vi "Power Output Find Pad Values.vi"(11 "Test Parameters":T1={"Stimulus"={"Frequency Type"=enum."Band Edges", "Frequency Ranges"=[], "TX 1 Frequency (MHz)"={"Min"=0.0, "Max"=0.0}, "TX 2 Frequency (MHz)"={"Min"=0.0, "Max"=0.0}, "RX Frequency (MHz)"={"Min"=0.0, "Max"=0.0}, "Pad Model Number"="", "Pad Serial Number"="", "Pad Values"=[]}, "Measurement"={"DUT Port"=enum."Port 1", "Direction"=0, "Frequency Step Size"=0}, "Display"={"Frequency"={"Min"=-1.0, "Max"=-1.0}, "Power"={"Min"=-1, "Max"=-1}}, "Limit"={"Min Power (dBm)"=44.0}, "Calibration"={"Calibrated?"=FALSE}} {"Measurement"."Frequency Step Size" items=["0.2", "0.4", "1.0", "2.0", "4.0"]; "Measurement"."Direction" items=["Reverse", "Forward", "Auxiliary"]}) -> (2 "Values Present?":bool, 3 "Pad Values Out":dbl[][](array[numeric]))   [LabVIEW 2011]
uses:
  TypeDefs/Power Output Test Parameters.ctl
  TypeDefs/Power Output Stimulus Parameters.ctl
  TypeDefs/Power Output Measurement Parameters.ctl
  BPIMCore EXT/HW IO/DUTport.ctl
  BPIMCore EXT/HW IO/MeasMode.ctl
  BPIMCore EXT/HW IO/PIM Sweep Step Size.ctl
  TypeDefs/Power Output Display Parameters.ctl
  TypeDefs/Power Output Limit Parameters.ctl
  TypeDefs/Power Output Calibration State.ctl
  Summitek EXT/OpenG EXT/array/array.llb/Filter 1D Array with Scalar (DBL)__ogtk.vi
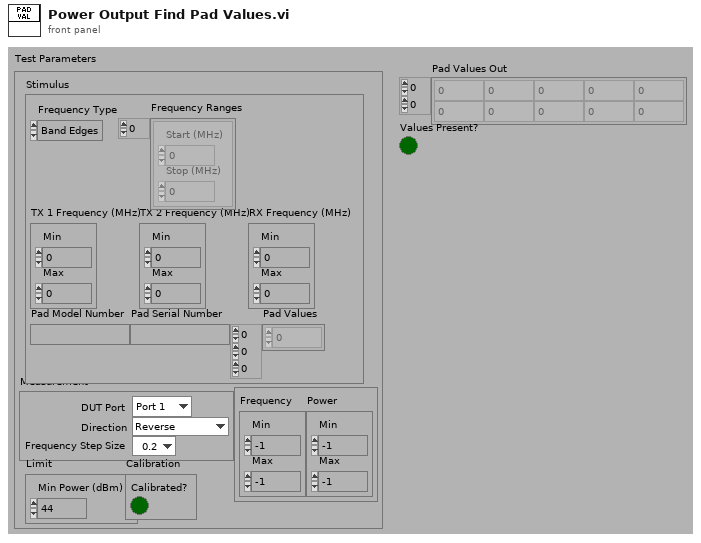
[diagram p1: front panel]
types:
  T1 = typedef "Power Output Test Parameters.ctl" = cluster{"Stimulus":T2, "Measurement":T3, "Display":T7, "Limit":T8, "Calibration":T9}
  T2 = typedef "Power Output Stimulus Parameters.ctl" = cluster{"Frequency Type":enum16{"Band Edges", "Custom"}, "Frequency Ranges":cluster{"Start (MHz)":dbl, "Stop (MHz)":dbl}[], "TX 1 Frequency (MHz)":cluster{"Min":dbl, "Max":dbl}, "TX 2 Frequency (MHz)":cluster{"Min":dbl, "Max":dbl}, "RX Frequency (MHz)":cluster{"Min":dbl, "Max":dbl}, "Pad Model Number":string, "Pad Serial Number":string, "Pad Values":dbl[][][]}
  T3 = typedef "Power Output Measurement Parameters.ctl" = cluster{"DUT Port":T4, "Direction":T5, "Frequency Step Size":T6}
  T4 = typedef "DUTport.ctl" = enum16{"Port 1", "Port 2"}
  T5 = typedef "MeasMode.ctl" = u16
  T6 = typedef "PIM Sweep Step Size.ctl" = u16
  T7 = typedef "Power Output Display Parameters.ctl" = cluster{"Frequency":cluster{"Min":dbl, "Max":dbl}, "Power":cluster{"Min":i32, "Max":i32}}
  T8 = typedef "Power Output Limit Parameters.ctl" = cluster{"Min Power (dBm)":dbl}
  T9 = typedef "Power Output Calibration State.ctl" = cluster{"Calibrated?":bool}
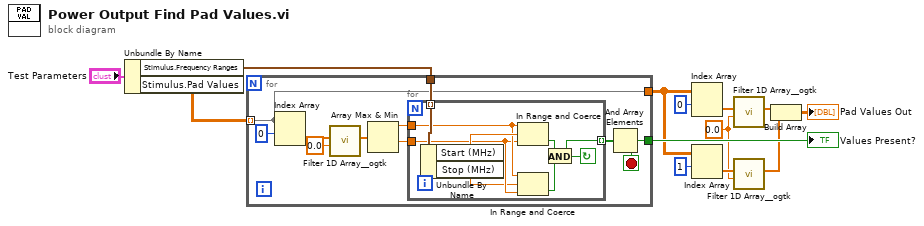
[diagram p0: block diagram]
diagram:
  w3 = 0.0
  n1 = Unbundle By Name("Test Parameters") -> ("Stimulus.Frequency Ranges"=w11:cluster{"Start (MHz)":dbl, "Stop (MHz)":dbl}[], "Stimulus.Pad Values"=w10:dbl[][][])
  n2 = for {
    tunnel: w10 -> [w14] mode=indexing
    tunnel: w11 -> [w22]
    tunnel: [w20] -> w13
    tunnel: [w14] -> w1
    stop <- w20 stop-if-true
    n3 = Index Array(array=w14, index (row)=0 ("disabled index (col)")) -> (element=w15:dbl[])  [unwired: 1 in]
    n4 = call-poly "Filter 1D Array__ogtk.vi"("items to filter"=0.0, "array"=w15) -> ("filtered array"=w16:dbl[])  [unwired: 4 in, 1 out]
    n5 = Array Max & Min(array=w16) -> (max value=w19:dbl, min value=w18:dbl)  [unwired: 2 out]
    n6 = for {
      tunnel: w22 -> [w31] mode=indexing
      tunnel: w19 -> [w29]
      tunnel: w18 -> [w28]
      tunnel: [w24] -> w21 mode=indexing
      stop <- w24 continue-if-true
      n7 = Unbundle By Name(w31) -> ("Start (MHz)"=w30:dbl, "Stop (MHz)"=w27:dbl)
      n8 = In Range and Coerce(upper limit=w29, x=w30, lower limit=w28) -> (In Range?=w25:bool)  [unwired: 1 out]
      n9 = In Range and Coerce(upper limit=w29, x=w27, lower limit=w28) -> (In Range?=w26:bool)  [unwired: 1 out]
      n10 = And(x=w25, y=w26) -> (x .and. y?=w24:bool)
    }
    n11 = And Array Elements(Boolean array=w21) -> (logical AND=w20:bool)
  }
  "Values Present?" <- w13
  n12 = Index Array(array=w1, index (row)=0 ("disabled index (col)")) -> (element=w9:dbl[])  [unwired: 1 in]
  n13 = Index Array(array=w1, index (row)=1 ("disabled index (col)")) -> (element=w6:dbl[])  [unwired: 1 in]
  n14 = call-poly "Filter 1D Array__ogtk.vi"("items to filter"=w3, "array"=w9) -> ("filtered array"=w5:dbl[])  [unwired: 4 in, 1 out]
  n15 = call-poly "Filter 1D Array__ogtk.vi"("items to filter"=w3, "array"=w6) -> ("filtered array"=w4:dbl[])  [unwired: 4 in, 1 out]
  n16 = Build Array(w5, w4) -> (→"Pad Values Out":dbl[][])
